vi "Get Active Functions.vi"(0 "functionbase in":refnum<class "functionbase.lvclass">, 11 "error in (no error)":errorcluster) -> (4 "functionbase out":refnum<class "functionbase.lvclass">, 6 "Syntax Index":i32, 15 "error out":errorcluster)   [LabVIEW 2019, in "LSL.lvlib" / "functionbase.lvclass"]
uses:
  functionbase.lvclass
  functionbase.lvclass/functionbase.ctl
  properties/Read Smart Syntax Representation.vi
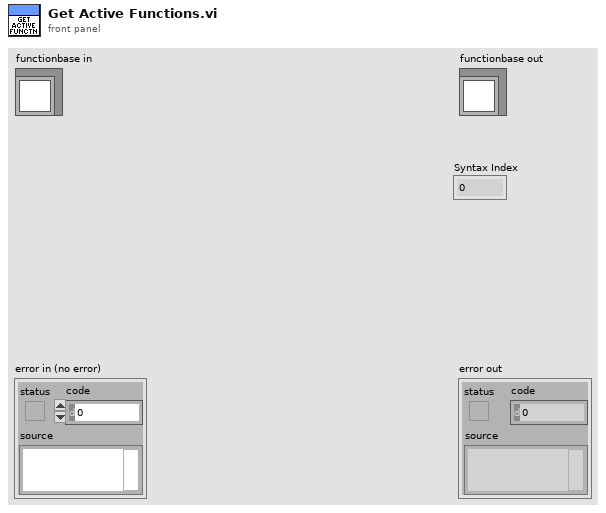
[diagram p1: front panel]
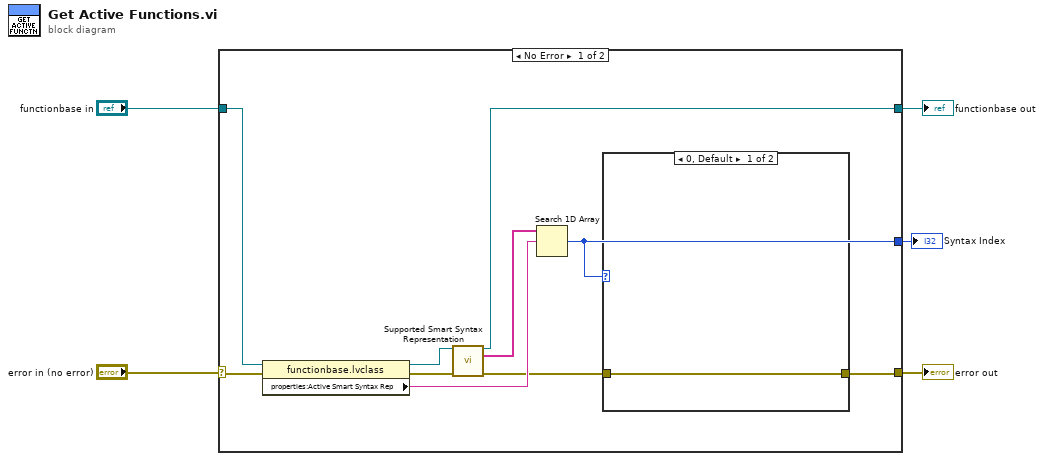
[diagram p0: block diagram]
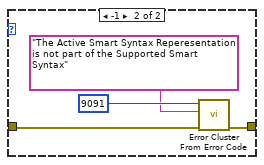
[diagram p2: hidden frame]
diagram:
  n1 = case shown="No Error" "error in (no error)" {
    selector: "error in (no error)" -> [w11 w22]
    tunnel: [w6 w22] -> w4
    tunnel: [w9 w21] -> w2
    tunnel: "functionbase in" -> [w10 w21]
    tunnel: [w8 _] -> w1
    frame No Error {
      n2 = property class="functionbase.lvclass"(reference=w10, error in=w11) -> (reference out=w14:refnum<class "functionbase.lvclass">, error out=w15:errorcluster, "properties:Active Smart Syntax Rep"=w12:string)
      n3 = call-dynamic "Supported Smart Syntax Representation.vi"("functionbase in"=w14, "error in (no error)"=w15) -> ("functionbase out"=w9:refnum<class "functionbase.lvclass">, "Smart Syntax Representation List"=w13:string[], "error out"=w7:errorcluster)  [unwired: 11 in]
      n4 = Search 1D Array(1D array=w13, element=w12) -> (index of element=w8:i32)  [unwired: 1 in]
      n5 = case shown="0, Default" w8 {
        tunnel: w7 -> [w16 w19]
        tunnel: [w16 w20] -> w6
        frame 0, Default {
        }
        frame -1 {
          n6 = call <vilib>:"Error Cluster From Error Code.vi"("error in (no error)"=w19, "error message (\"\")"="The Active Smart Syntax Reperesentation is not part of the Supported Smart Syntax" ("error message (\"\")"), "error code (0)"=9091) -> ("error out"=w20:errorcluster)  [unwired: 6 in]
        }
      }
    }
    frame Error {
    }
  }
  "error out" <- w4
  "functionbase out" <- w2
  "Syntax Index" <- w1
